vi "Origin_XY_2nd.vi"(0 "PortNumber":u8=11) -> (1 "Received String1":string="OK\r\n", 2 "Received String2":string="R\r\n", 3 "OK Done":bool=TRUE)   [LabVIEW 2013]
panel:
  # "Port Number 0=COM1"
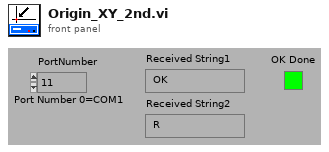
[diagram p1: front panel]
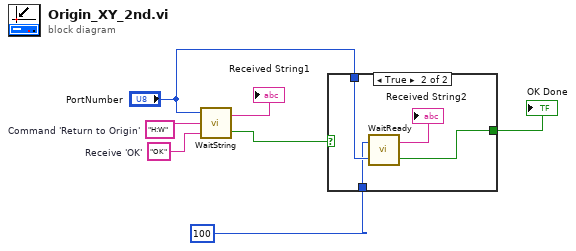
[diagram p0: block diagram]
diagram:
  w5 = "OK"  # Receive 'OK'
  w6 = "H:W"  # Command 'Return to Origin'
  n1 = call "WaitString.vi"("String to Receive"=w5, "String to Send"=w6, "PortNumber"="PortNumber") -> ("OK Done"=w1:bool, "String Received"=→"Received String1":string)
  n2 = case shown="True" w1 {
    selector: w1 -> [w8 _]
    tunnel: "PortNumber" -> [_ w12]
    tunnel: [w8 w10] -> w4
    tunnel: 100 -> [_ w9]
    frame False {
    }
    frame True {
      n3 = call "WaitReady.vi"("PortNumber"=w12, "Residence time in ms"=w9) -> ("OK Done"=w10:bool, "String Received"=→"Received String2":string)
    }
  }
  "OK Done" <- w4
